vi "Move Data.vi"(5 "Copy Data? [T]":bool=TRUE, 7 "Copy Paths? [T]":bool=TRUE, 8 "error in (no error)":errorcluster, 10 "Carya Config source":refnum<class "Carya Config.lvclass">, 11 "Carya Config dest":refnum<class "Carya Config.lvclass">) -> (0 "error out":errorcluster, 3 "Carya Config out":refnum<class "Carya Config.lvclass">)   [LabVIEW 2013, in "Carya Config.lvclass"]
doc: "Copyright 2018, Carya Automatisering, Wiebe Walstra."
uses:
  Carya Config.lvclass
  Carya Config.lvclass/Carya Config.ctl
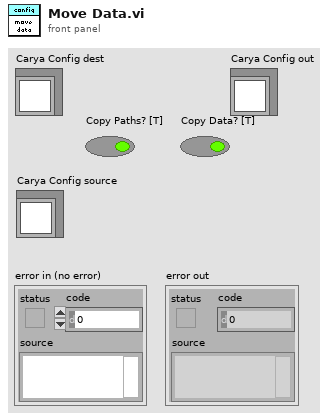
[diagram p1: front panel]
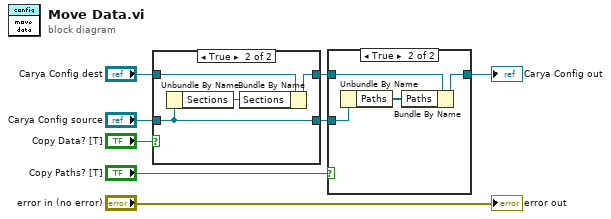
[diagram p0: block diagram]
diagram:
  n1 = case shown="True" "Copy Data? [T]" {
    tunnel: "Carya Config source" -> [w10 w11]
    tunnel: "Carya Config dest" -> [w9 w14]
    tunnel: [w9 w13] -> w7
    tunnel: [w10 w11] -> w5
    frame False {
    }
    frame True {
      n2 = Unbundle By Name(w11) -> ("Sections"=w12:refnum<class "CConfig Object.lvclass">)
      n3 = Bundle By Name(cluster=w14, "Sections"=w12) -> (w13:refnum<class "Carya Config.lvclass">)
    }
  }
  n4 = case shown="True" "Copy Paths? [T]" {
    tunnel: w7 -> [w15 w19]
    tunnel: [w15 w18] -> w6
    tunnel: w5 -> [_ w16]
    frame False {
    }
    frame True {
      n5 = Unbundle By Name(w16) -> ("Paths"=w17:path[])
      n6 = Bundle By Name(cluster=w19, "Paths"=w17) -> (w18:refnum<class "Carya Config.lvclass">)
    }
  }
  "Carya Config out" <- w6
  "error out" <- "error in (no error)"
